vi "Calculate.vi"(8 "error in (no error)":errorcluster, 10 "Async Settings":T1 {"Frames"."Protection Configurations"."CRC Channels"."Data Type" items=["Signed", "Unsigned", "IEEE Float"]}, 11 "Data Refs":T7) -> (0 "error out":errorcluster, 2 "Async Settings":T1 {"Frames"."Protection Configurations"."CRC Channels"."Data Type" items=["Signed", "Unsigned", "IEEE Float"]})   [LabVIEW 2015, in "Protection and Rolling Counter Addon Engine.lvlib"]
uses:
  Protection and Rolling Counter Addon Engine.lvlib
  Types/RT Async Engine Variables.ctl
  Types/RT Frame Settings.ctl
  Types/RT Protection Configuration.ctl
  Shared/Types/Protection Type.ctl
  Shared/Types/InputChannelConfiguration.ctl
  Types/RT Counter Settings.ctl
  Types/RT Data References.ctl
  <vilib>/NI/NIVS Inline Async API/_Data Access Engine/Data Access Engine/Types/Write.DVR.ctl
  <vilib>/NI/NIVS Inline Async API/_Data Access Engine/Access Type Classes/Write/Write.lvclass
  <vilib>/NI/NIVS Inline Async API/_Data Access Engine/Data Access Engine/Types/Read.DVR.ctl
  <vilib>/NI/NIVS Inline Async API/_Data Access Engine/Access Type Classes/Read/Read.lvclass
  <vilib>/NI/NIVS Inline Async API/_Data Access Engine/Access Type Classes/Read/Read.lvclass/Read.ctl
  <vilib>/NI/NIVS Inline Async API/_Data Access Engine/Access Type Classes/Write/Write.lvclass/Write.ctl
  <vilib>/NI/NIVS Inline Async API/_Data Access Engine/Data Access Engine/Methods/Read.Data.vi
  <vilib>/NI/NIVS Inline Async API/_Data Access Engine/Data Access Engine/Methods/Write.Data.Buffer.vi
  <vilib>/NI/NIVS Inline Async API/_Data Access Engine/Data Access Engine/Methods/Write.Data.Commit.vi
  <vilib>/NI/NIVS Inline Async API/_Data Access Engine/Data Access Engine/Methods/Write.Data.vi
  <vilib>/NI/NIVS Inline Async API/_Data Access Engine/Access Type Classes/Read/Read.ProcessData.vi
  <vilib>/NI/NIVS Inline Async API/_Data Access Engine/Access Type Classes/Write/Write.Buffer.vi
  <vilib>/NI/NIVS Inline Async API/_Data Access Engine/Access Type Classes/Write/Write.Commit.vi
  <vilib>/NI/NIVS Inline Async API/_Data Access Engine/Access Type Classes/Write/Write.ProcessData.vi
  <vilib>/xnet/xnet.llb/XNET Convert (Signal to Frame Raw).vi
  <vilib>/xnet/xnet.llb/XNET Convert (Signal to Frame CAN).vi
  <vilib>/xnet/xnet.llb/XNET Write (Frame CAN).vi
  <vilib>/NI/NIVS Inline Async API/_Data Access Engine/Data Access Engine/Data Access Engine.lvclass
  Shared/Protection and Rolling Counter Addon Shared.lvlib
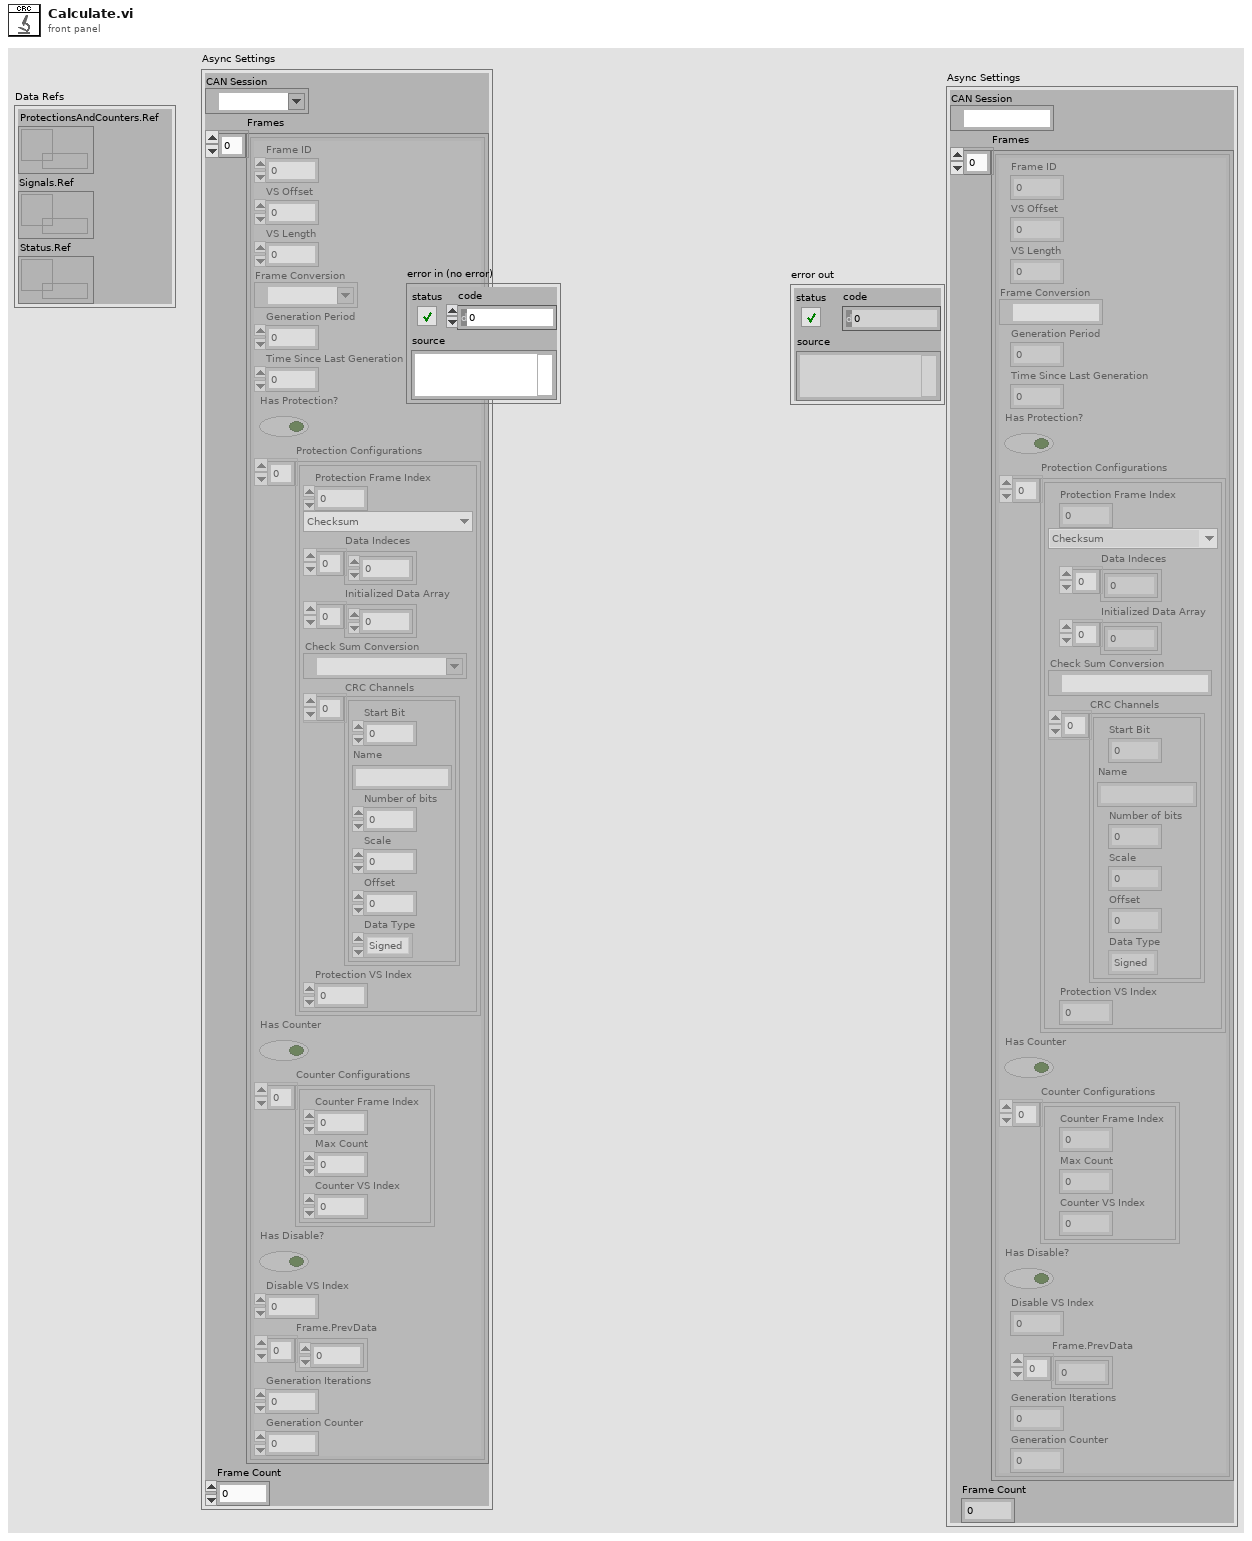
[diagram p1: front panel]
types:
  T1 = typedef "Protection and Rolling Counter Addon Engine.lvlib/RT Async Engine Variables.ctl" = cluster{"CAN Session":refnum<k21>, "Frames":T2[], "Frame Count":i32}
  T2 = typedef "Protection and Rolling Counter Addon Engine.lvlib/RT Frame Settings.ctl" = cluster{"Frame ID":u32, "VS Offset":i32, "VS Length":i32, "Frame Conversion":refnum<k21>, "Generation Period":u32, "Time Since Last Generation":u32, "Has Protection?":bool, "Protection Configurations":T3[], "Has Counter":bool, "Counter Configurations":T6[], "Has Disable?":bool, "Disable VS Index":i32, "Frame.PrevData":dbl[], "Generation Iterations":u32, "Generation Counter":u32}
  T3 = typedef "Protection and Rolling Counter Addon Engine.lvlib/RT Protection Configuration.ctl" = cluster{"Protection Frame Index":i32, "Protection Type":T4, "Data Indeces":i32[], "Initialized Data Array":dbl[], "Check Sum Conversion":refnum<k21>, "CRC Channels":T5[], "Protection VS Index":i32}
  T4 = typedef "Protection and Rolling Counter Addon Shared.lvlib/Protection Type.ctl" = enum16{"Checksum", "CRC"}
  T5 = typedef "Protection and Rolling Counter Addon Shared.lvlib/InputChannelConfiguration.ctl" = cluster{"Start Bit":i32, "Name":string, "Number of bits":i32, "Scale":dbl, "Offset":dbl, "Data Type":u32}
  T6 = typedef "Protection and Rolling Counter Addon Engine.lvlib/RT Counter Settings.ctl" = cluster{"Counter Frame Index":i32, "Max Count":dbl, "Counter VS Index":i32}
  T7 = typedef "Protection and Rolling Counter Addon Engine.lvlib/RT Data References.ctl" = cluster{"ProtectionsAndCounters.Ref":T8, "Signals.Ref":T9, "Status.Ref":T8}
  T8 = typedef "Data Access Engine.lvlib/Data Access Engine.lvclass/Write.DVR.ctl" = refnum<data-value>
  T9 = typedef "Data Access Engine.lvlib/Data Access Engine.lvclass/Read.DVR.ctl" = refnum<data-value>
  T10 = typedef "XNET Frame CAN.ctl" = cluster{"timestamp":timestamp, "payload":u8[], "identifier":u32, "type":T11, "extended?":bool, "echo?":bool}
  T11 = typedef "XNET Frame Type CAN.ctl" = u8
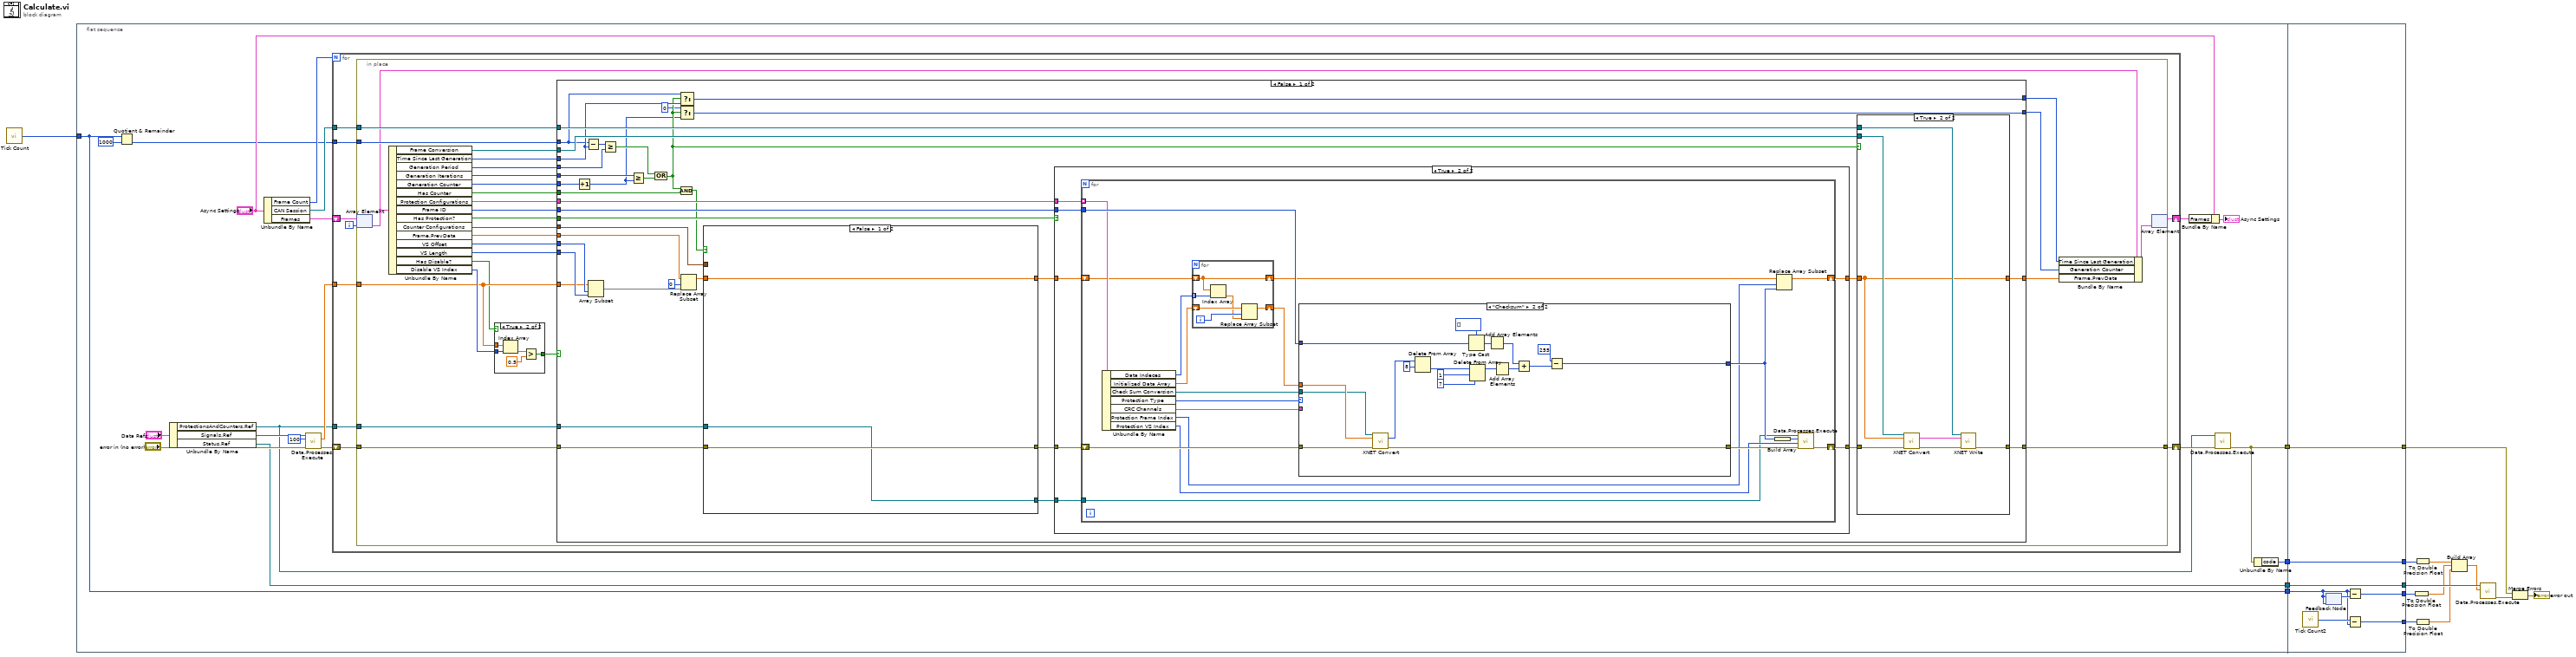
[diagram p0: block diagram]
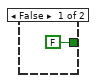
[diagram p2: hidden frame]
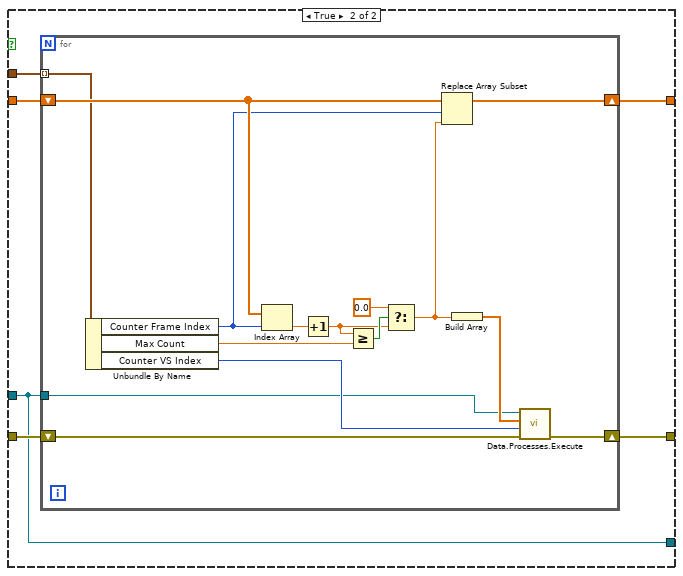
[diagram p3: hidden frame]
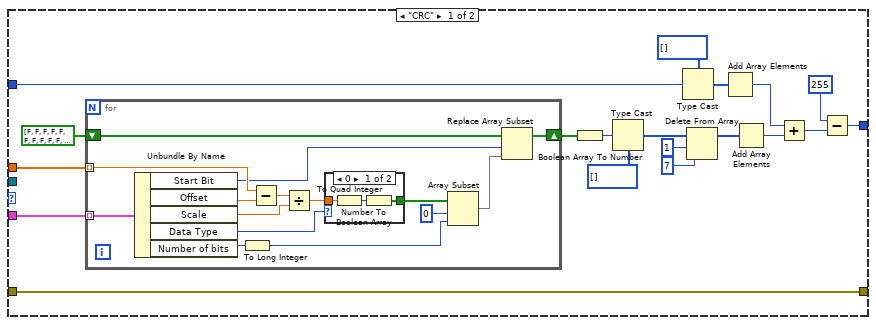
[diagram p5: hidden frame]
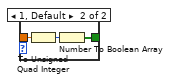
[diagram p6: hidden frame]
diagram:
  n1 = call "Tick Count"() -> ("Tick Count(uSec)"=w16:u32)
  n2 = flat-sequence {
    tunnel: w16 -> [w20]
    tunnel: [w18] -> w9
    tunnel: [w22] -> w8
    tunnel: [w20] -> w7
    tunnel: [w17] -> w4
    tunnel: [w249] -> w14
    tunnel: [w251] -> w15
    tunnel: [w252] -> w11
    tunnel: w9 -> [w252]
    tunnel: w8 -> [w251]
    tunnel: w7 -> [w247]
    tunnel: [w246] -> w6
    tunnel: [w245] -> w5
    tunnel: w4 -> [w245]
    frame #0 {
      n3 = Quotient & Remainder(x=w20, y=u32 1000) -> (floor(x/y)=w21:u32)  [unwired: 1 out]
      n4 = Unbundle By Name("Data Refs") -> ("ProtectionsAndCounters.Ref"=w27:T8, "Signals.Ref"=w33:T9, "Status.Ref"=w22:T8)
      n5 = Unbundle By Name("Async Settings") -> ("Frame Count"=w26:i32, "CAN Session"=w36:refnum<k21>, "Frames"=w35:T2[])
      n6 = call-poly <vilib>:"Data.Processes.Execute.vi"("error in (no error)"="error in (no error)", "timeout ms"=100, "Ref"=w33) -> ("error out"=w30:errorcluster, "Values"=w29:dbl[])  [unwired: 6 in, 1 out]
      n7 = for {
        N: w26 -> [_]
        tunnel: w29 -> [w42]
        shift-right: [w44] -> w28
        shift-left: w30 -> [w45]
        tunnel: w21 -> [w43]
        tunnel: w36 -> [w41]
        tunnel: w27 -> [w40]
        shift-right: [w37] -> w24
        shift-left: w35 -> [w39]
        i -> [w38]
        n8 = in-place {
          in-place-border: w45 -> [w72]
          in-place-border: [w71] -> w44
          in-place-border: w43 -> [w67]
          in-place-border: w42 -> [w63]
          in-place-border: w41 -> [w60]
          in-place-border: w40 -> [w57]
          n9 = in-place-array #1(w39, w38) -> (w47:T2)
          n10 = Unbundle By Name(w47) -> ("Frame Conversion"=w65:refnum<k21>, "Time Since Last Generation"=w58:u32, "Generation Period"=w59:u32, "Generation Iterations"=w50:u32, "Generation Counter"=w49:u32, "Has Counter"=w68:bool, "Protection Configurations"=w56:T3[], "Frame ID"=w55:u32, "Has Protection?"=w54:bool, "Counter Configurations"=w66:T6[], "Frame.PrevData"=w53:dbl[], "VS Offset"=w70:i32, "VS Length"=w69:i32, "Has Disable?"=w62:bool, "Disable VS Index"=w64:i32)
          n11 = case shown="True" w62 {
            tunnel: w64 -> [_ w78]
            tunnel: w63 -> [_ w77]
            tunnel: [FALSE w75] -> w61
            frame False {
            }
            frame True {
              n12 = Index Array(array=w77, index=w78) -> (element=w76:dbl)
              n13 = Greater?(x=w76, y=0.5 ("x")) -> (0:w75:bool)
            }
          }
          n14 = case shown="False" w61 {
            tunnel: w72 -> [w98 w244]
            tunnel: [w114 w244] -> w71
            tunnel: w70 -> [w113 _]
            tunnel: w69 -> [w112 _]
            tunnel: w68 -> [w111 _]
            tunnel: w67 -> [w88 _]
            tunnel: w59 -> [w100 _]
            tunnel: w66 -> [w110 _]
            tunnel: w56 -> [w108 _]
            tunnel: w54 -> [w107 _]
            tunnel: w55 -> [w106 _]
            tunnel: w65 -> [w104 _]
            tunnel: w63 -> [w103 w243]
            tunnel: w60 -> [w102 _]
            tunnel: w58 -> [w89 w242]
            tunnel: w57 -> [w96 _]
            tunnel: w53 -> [w94 _]
            tunnel: [w90 w243] -> w52
            tunnel: [w87 w242] -> w51
            tunnel: w50 -> [w85 _]
            tunnel: w49 -> [w86 w241]
            tunnel: [w79 w241] -> w48
            frame False {
              n15 = Increment(x=w86) -> (x+1=w81:u32)
              n16 = Subtract(x=w88, y=w89) -> (x-y=w101:u32)
              n17 = Array Subset(array=w103, index=w113, length=w112) -> (w92:dbl[])
              n18 = Greater Or Equal?(x=w101, y=w100) -> (x >= y?=w83:bool)
              n19 = Greater Or Equal?(x=w85, y=w81) -> (x >= y?=w84:bool)
              n20 = Compound Arithmetic op=OR(w83, w84) -> (w82:bool)
              n21 = Select(t=w88, s=w82, f=w89) -> (s? t:f=w87:u32)
              n22 = Select(t=u32 0, s=w82, f=w81) -> (s? t:f=w79:u32)
              n23 = Compound Arithmetic op=AND(w82, w111) -> (w99:bool)
              n24 = Replace Array Subset(array=w94, new element=w92, index=0) -> (w91:dbl[])
              n25 = case shown="False" w99 {
                tunnel: w91 -> [w118 w124]
                tunnel: [w118 w123] -> w109
                tunnel: w110 -> [_ w122]
                tunnel: w98 -> [w117 w121]
                tunnel: [w117 w120] -> w97
                tunnel: w96 -> [w116 w119]
                tunnel: [w116 w119] -> w95
                frame False {
                }
                frame True {
                  n26 = for {
                    shift-right: [w137] -> w123
                    shift-left: w124 -> [w139]
                    tunnel: w122 -> [w136] mode=indexing
                    shift-right: [w126] -> w120
                    shift-left: w121 -> [w127]
                    tunnel: w119 -> [w125]
                    n27 = Unbundle By Name(w136) -> ("Counter Frame Index"=w132:i32, "Max Count"=w138:dbl, "Counter VS Index"=w130:i32)
                    n28 = Index Array(array=w139, index=w132) -> (element=w133:dbl)
                    n29 = Increment(x=w133) -> (x+1=w131:dbl)
                    n30 = Greater Or Equal?(x=w131, y=w138) -> (x >= y?=w135:bool)
                    n31 = Select(t=0.0, s=w135, f=w131) -> (s? t:f=w129:dbl)
                    n32 = Replace Array Subset(array=w139, new element=w129, index=w132) -> (w137:dbl[])
                    n33 = Build Array(w129) -> (w128:dbl[])
                    n34 = call-poly <vilib>:"Data.Processes.Execute.vi"("error in (no error)"=w127, "Offset"=w130, "Values"=w128, "Ref"=w125) -> ("error out"=w126:errorcluster)  [unwired: 7 in]
                  }
                }
              }
              n35 = case shown="True" w107 {
                tunnel: w106 -> [_ w148]
                tunnel: w97 -> [w141 w147]
                tunnel: [w141 w146] -> w115
                tunnel: w109 -> [w140 w145]
                tunnel: w108 -> [_ w144]
                tunnel: [w140 w143] -> w105
                tunnel: w95 -> [_ w142]
                frame False {
                }
                frame True {
                  n36 = for {
                    tunnel: w148 -> [w167]
                    tunnel: w144 -> [w164] mode=indexing
                    shift-right: [w156] -> w146
                    shift-left: w147 -> [w166]
                    shift-right: [w165] -> w143
                    shift-left: w145 -> [w161]
                    tunnel: w142 -> [w149]
                    n37 = Unbundle By Name(w164) -> ("Data Indeces"=w162:i32[], "Initialized Data Array"=w159:dbl[], "Check Sum Conversion"=w151:refnum<k21>, "Protection Type"=w152:T4, "CRC Channels"=w163:T5[], "Protection Frame Index"=w150:i32, "Protection VS Index"=w153:i32)
                    n38 = for {
                      shift-right: [w172] -> w160
                      shift-left: w161 -> [w172]
                      tunnel: w162 -> [w173] mode=indexing
                      shift-right: [w168] -> w158
                      shift-left: w159 -> [w171]
                      i -> [w170]
                      n39 = Index Array(array=w172, index=w173) -> (element=w169:dbl)
                      n40 = Replace Array Subset(array=w171, new element=w169, index=w170) -> (w168:dbl[])
                    }
                    n41 = case shown="\"Checksum\"" w152 {
                      tunnel: w167 -> [w186 w225]
                      tunnel: [w181 w220] -> w155
                      tunnel: w166 -> [w177 w219]
                      tunnel: [w177 w218] -> w157
                      tunnel: w163 -> [w175 _]
                      tunnel: w158 -> [w176 w215]
                      tunnel: w151 -> [_ w214]
                      frame "CRC" {
                        n42 = for {
                          tunnel: w175 -> [w207] mode=indexing
                          shift-right: [w198] -> w180
                          shift-left: bool[] [FALSE, FALSE, FALSE, FALSE, FALSE, FALSE, FALSE, FALSE, FALSE, FALSE, FALSE, FALSE, FALSE, FALSE, FALSE, FALSE, FALSE, FALSE, FALSE, FALSE, FALSE, FALSE, FALSE, FALSE, FALSE, FALSE, FALSE, FALSE, FALSE, FALSE, FALSE, FALSE, FALSE, FALSE, FALSE, FALSE, FALSE, FALSE, FALSE, FALSE, FALSE, FALSE, FALSE, FALSE, FALSE, FALSE, FALSE, FALSE, FALSE, FALSE, FALSE, FALSE, FALSE, FALSE, FALSE, FALSE, FALSE, FALSE, FALSE, FALSE, FALSE, FALSE, FALSE, FALSE] ("Boolean array") -> [w200]
                          tunnel: w176 -> [w197] mode=indexing
                          n43 = Unbundle By Name(w207) -> ("Start Bit"=w194:i32, "Offset"=w206:dbl, "Scale"=w204:dbl, "Data Type"=w196:u32, "Number of bits"=w202:i32)
                          n44 = To Long Integer(number=w202) -> (32bit integer=w193:i32)
                          n45 = Subtract(x=w197, y=w206) -> (x-y=w205:dbl)
                          n46 = Divide(x=w205, y=w204) -> (x/y=w203:dbl)
                          n47 = case shown="0" w196 {
                            tunnel: w203 -> [w210 w213]
                            tunnel: [w208 w211] -> w195
                            frame 0 {
                              n48 = To Quad Integer(1:w210) -> (0:w209:i64)
                              n49 = Number To Boolean Array(number=w209) -> (Boolean array=w208:bool[])
                            }
                            frame 1, Default {
                              n50 = To Unsigned Quad Integer(1:w213) -> (0:w212:u64)
                              n51 = Number To Boolean Array(number=w212) -> (Boolean array=w211:bool[])
                            }
                          }
                          n52 = Array Subset(array=w195, index=0, length=w193) -> (w199:bool[])
                          n53 = Replace Array Subset(array=w200, new element=w199, index=w194) -> (w198:bool[])
                        }
                        n54 = Boolean Array To Number(Boolean array=w180) -> (number=w179:u64)
                        n55 = Type Cast(type=u8[] [], x=w179) -> (*(type *) &x=w192:u8[])
                        n56 = Type Cast(type=u8[] [], x=w186) -> (*(type *) &x=w185:u8[])
                        n57 = Delete From Array(array=w192, length=1, index=7) -> (array with subset deleted=w189:u8[])  [unwired: 1 out]
                        n58 = Add Array Elements(numeric array=w185) -> (sum=w184:u8)
                        n59 = Add Array Elements(numeric array=w189) -> (sum=w188:u8)
                        n60 = Add(x=w184, y=w188) -> (x+y=w183:u8)
                        n61 = Subtract(x=u8 255, y=w183) -> (x-y=w181:u8)
                      }
                      frame "Checksum" {
                        n62 = call-poly <vilib>:"XNET Convert.vi"("session in"=w214, "signal data"=w215, "error in (no error)"=w219) -> ("frame data"=w216:u8[], "error out"=w218:errorcluster)  [unwired: 10 in, 1 out]
                        n63 = Delete From Array(array=w216, length=8) -> (deleted portion=w231:u8[])  [unwired: 1 in, 1 out]
                        n64 = Type Cast(type=u8[] [], x=w225) -> (*(type *) &x=w224:u8[])
                        n65 = Delete From Array(array=w231, length=1, index=7) -> (array with subset deleted=w228:u8[])  [unwired: 1 out]
                        n66 = Add Array Elements(numeric array=w224) -> (sum=w223:u8)
                        n67 = Add Array Elements(numeric array=w228) -> (sum=w227:u8)
                        n68 = Add(x=w223, y=w227) -> (x+y=w222:u8)
                        n69 = Subtract(x=u8 255, y=w222) -> (x-y=w220:u8)
                      }
                    }
                    n70 = Build Array(w155) -> (w154:u8[])
                    n71 = Replace Array Subset(array=w160, new element=w155, index=w150) -> (w165:dbl[])
                    n72 = call-poly <vilib>:"Data.Processes.Execute.vi"("error in (no error)"=w157, "Offset"=w153, "Values"=w154, "Ref"=w149) -> ("error out"=w156:errorcluster)  [unwired: 7 in]
                  }
                }
              }
              n73 = case shown="True" w82 {
                tunnel: w115 -> [w233 w239]
                tunnel: [w233 w237] -> w114
                tunnel: w105 -> [w232 w234]
                tunnel: w104 -> [_ w236]
                tunnel: w102 -> [_ w235]
                tunnel: [w232 w234] -> w90
                frame False {
                }
                frame True {
                  n74 = call-poly <vilib>:"XNET Convert.vi"("session in"=w236, "signal data"=w234, "error in (no error)"=w239) -> ("frame data"=w240:T10[], "error out"=w238:errorcluster)  [unwired: 9 in, 2 out]
                  n75 = call-poly <vilib>:"XNET Write.vi"("session in"=w235, "data"=w240, "error in (no error)"=w238) -> ("error out"=w237:errorcluster)  [unwired: 11 in, 1 out]
                }
              }
            }
            frame True {
            }
          }
          n76 = Bundle By Name(cluster=w47, "Time Since Last Generation"=w51, "Generation Counter"=w48, "Frame.PrevData"=w52) -> (w46:T2)
          n77 = in-place-array #1(w46) -> (w37:T2[])  [unwired: 1 out]
        }
      }
      n78 = Bundle By Name(cluster="Async Settings", "Frames"=w24) -> (→"Async Settings":T1)
      n79 = call-poly <vilib>:"Data.Processes.Execute.vi"("error in (no error)"=w28, "Ref"=w27) -> ("error out"=w18:errorcluster)  [unwired: 9 in]
      n80 = Unbundle By Name(w18) -> ("code"=w17:i32)
    }
    frame #1 {
      n81 = call "Tick Count2"() -> ("Tick Count(uSec)"=w248:u32)
      n82 = feedback #2(w247) -> (w250:u32)
      n83 = feedback-in #2(w247) -> ()
      n84 = Subtract(x=w247, y=w250) -> (x-y=w249:u32)
      n85 = Subtract(x=w248, y=w247) -> (x-y=w246:u32)
    }
  }
  n86 = To Double Precision Float(number=w14) -> (double precision float=w2:dbl)
  n87 = To Double Precision Float(number=w5) -> (double precision float=w3:dbl)
  n88 = To Double Precision Float(number=w6) -> (double precision float=w1:dbl)
  n89 = Build Array(w3, w2, w1) -> (w13:dbl[])
  n90 = call-poly <vilib>:"Data.Processes.Execute.vi"("Values"=w13, "Ref"=w15) -> ("error out"=w12:errorcluster)  [unwired: 9 in]
  n91 = Merge Errors(w11, w12) -> (→"error out":errorcluster)
